vi "parse_solve_position_ik_resp_roslv.vi"(4 "error in":errorcluster, 7 "msg in":string) -> (0 "error out":errorcluster, 1 "IK Reply":T1, 2 "error byte":u8, 3 "msg out":string)   [LabVIEW 2014]
doc: "Parses a message into a solve postion for inverse kinematics"
uses:
  std_msgs/subs/parse_u8_scalar_roslv.vi
  std_msgs/subs/parse_float64_array_roslv.vi
  std_msgs/subs/parse_string_array_roslv.vi
  std_msgs/subs/parse_bool_array_roslv.vi
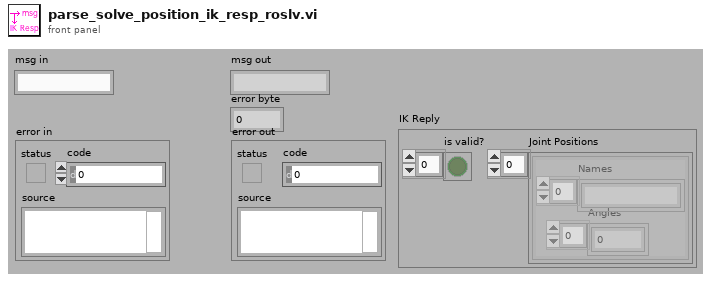
[diagram p1: front panel]
types:
  T1 = cluster{"is valid?":bool[], "Joint Positions":cluster{"Angles":dbl[], "Names":string[]}[]}
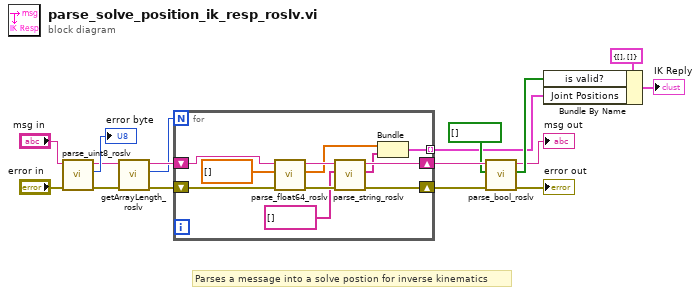
[diagram p0: block diagram]
diagram:
  # "Parses a message into a solve postion for inverse kinematics"
  n1 = call-poly "parse_uint8_roslv.vi"("error in"="error in", "msg in"="msg in") -> ("error out"=w3:errorcluster, "number"=→"error byte":u8, "msg out"=w15:string)  [unwired: 3 in]
  n2 = call "getArrayLength_roslv.vi"("error in"=w3, "msg in"=w15) -> ("error out"=w2:errorcluster, "array length"=w13:u32, "msg out"=w14:string)  [unwired: 3 in]
  n3 = for {
    N: w13 -> [_]
    shift-right: [w26] -> w12
    shift-left: w14 -> [w28]
    shift-right: [w23] -> w11
    shift-left: w2 -> [w22]
    tunnel: [w18] -> w7 mode=indexing
    n4 = call-poly "parse_float64_roslv.vi"("error in"=w22, "type"=dbl[] [], "msg in"=w28) -> ("error out"=w24:errorcluster, "number"=w20:dbl[], "msg out"=w27:string)  [unwired: 2 in]
    n5 = call-poly "parse_string_roslv.vi"("error in"=w24, "type"=string[] [], "msg in"=w27) -> ("error out"=w23:errorcluster, "strings"=w19:string[], "msg out"=w26:string)  [unwired: 2 in]
    n6 = Bundle("number"=w20, "strings"=w19) -> (w18:cluster{"number":dbl[], "strings":string[]})  [unwired: 1 in]
  }
  n7 = call-poly "parse_bool_roslv.vi"("error in"=w11, "type"=bool[] [], "msg in"=w12) -> ("error out"=→"error out":errorcluster, "boolean array"=w8:bool[], "msg out"=→"msg out":string)  [unwired: 2 in]
  n8 = Bundle By Name(cluster=T1 {"is valid?"=[], "Joint Positions"=[]} ("IK Reply"), "is valid?"=w8, "Joint Positions"=w7) -> (→"IK Reply":T1)
